vi "CoerceSelection.vi"(8 "error in (no error)":errorcluster, 11 "SetList Table ref":refnum<vi>) -> (0 "error out":errorcluster)   [LabVIEW 2013]
doc: "Corece table cells selection to be within table data bounds."
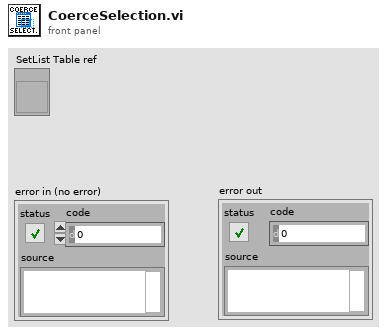
[diagram p1: front panel]
types:
  T1 = typedef "LVRowAndColumnTypeDef.ctl" = cluster{"Row":i32, "Column":i32}
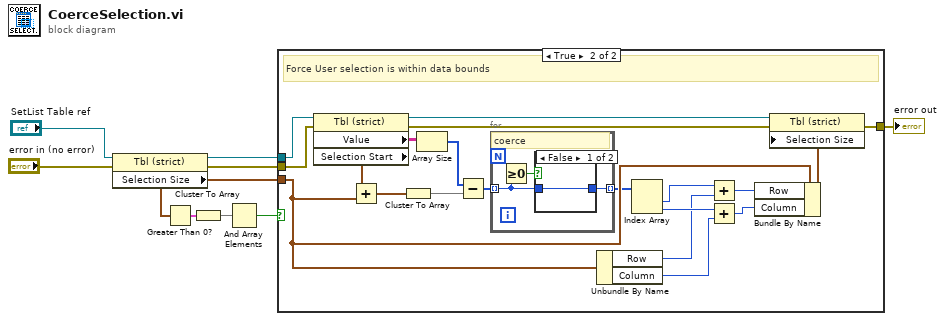
[diagram p0: block diagram]
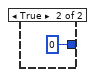
[diagram p3: hidden frame]
diagram:
  n1 = property class="Tbl (strict)"(reference="SetList Table ref", error in="error in (no error)") -> (reference out=w6:refnum<vi>, error out=w5:errorcluster, "Selection Size"=w4:T1)
  n2 = Greater Than 0?(x=w4) -> (x > 0?=w9:cluster{"Row":bool, "Column":bool})
  n3 = Cluster To Array(cluster=w9) -> (array=w8:bool[])
  n4 = And Array Elements(Boolean array=w8) -> (logical AND=w7:bool)
  n5 = case shown="True" w7 {
    tunnel: w6 -> [_ w30]
    tunnel: w5 -> [w10 w29]
    tunnel: w4 -> [_ w21]
    tunnel: [w10 w11] -> w2
    frame False {
      # "no selection, do nothing."
    }
    frame True {
      # "Force User selection is within data bounds"
      n6 = property class="Tbl (strict)"(reference=w30, error in=w29) -> (reference out=w25:refnum<vi>, error out=w24:errorcluster, "Value"=w27:string[][], "Selection Start"=w28:T1)
      n7 = Add(x=w28, y=w21) -> (x+y=w26:T1)
      n8 = Cluster To Array(cluster=w26) -> (array=w12:i32[])
      n9 = Array Size(array=w27) -> (size(s)=w13:i32[])
      n10 = Subtract(x=w13, y=w12) -> (x-y=w22:i32[])
      n11 = for {
        tunnel: w22 -> [w31] mode=indexing
        tunnel: [w32] -> w20 mode=indexing
        # "coerce"
        n12 = Greater Or Equal To 0?(x=w31) -> (x >= 0?=w33:bool)
        n13 = case shown="False" w33 {
          tunnel: [w34 0] -> w32
          tunnel: w31 -> [w34 _]
          frame False {
          }
          frame True {
          }
        }
      }
      n14 = Unbundle By Name(w21) -> ("Row"=w14:i32, "Column"=w15:i32)
      n15 = Index Array(array=w20) -> (element #1=w17:i32, element #2=w16:i32)  [unwired: 2 in]
      n16 = Add(x=w17, y=w14) -> (x+y=w19:i32)
      n17 = Add(x=w16, y=w15) -> (x+y=w18:i32)
      n18 = Bundle By Name(cluster=w21, "Row"=w19, "Column"=w18) -> (w23:T1)
      n19 = property class="Tbl (strict)"(reference=w25, error in=w24, "Selection Size"=w23) -> (error out=w11:errorcluster)  [unwired: 1 out]
    }
  }
  "error out" <- w2
